vi "P9P14T_Queue_Commands.vi"(1 "P9/P14-Magnet-Control":T1 {"Approach" items=["Linear", "NoOvershoot", "Oscillate"]}, 2 "P9/P14-Magnet-Control old status":T1 {"Approach" items=["Linear", "NoOvershoot", "Oscillate"]}, 3 "16T Queue":refnum<queue>) -> (0 "P9/P14-Magnet-Control new status":T1 {"Approach" items=["Linear", "NoOvershoot", "Oscillate"]})   [LabVIEW 2019]
uses:
  PPMS/P9P14_Magnet_Control.ctl
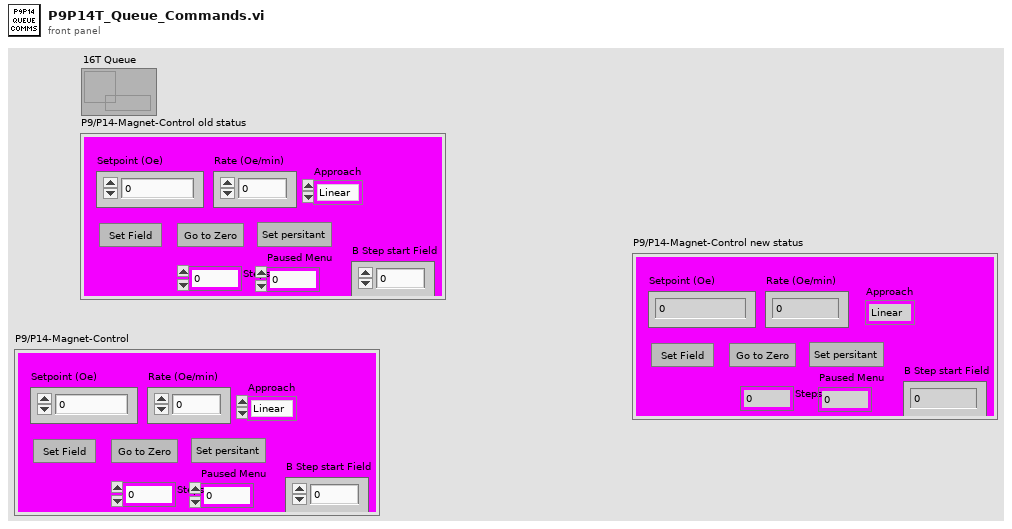
[diagram p1: front panel]
types:
  T1 = typedef "P9P14_Magnet_Control.ctl" = cluster{"Setpoint (Oe)":dbl, "Rate (Oe/min)":dbl, "Set Field":bool, "Go to zero":bool, "Set Persitant/non-pers":bool, "Approach":i32, "Steps":dbl, "Paused Menu":dbl, "B Step start Field":dbl}
  T2 = cluster{"Setpoint (Oe)":bool, "Rate (Oe/min)":bool, "Set Field":bool, "Go to zero":bool, "Set Persitant/non-pers":bool, "Approach":bool, "Steps":bool, "Paused Menu":bool, "B Step start Field":bool}
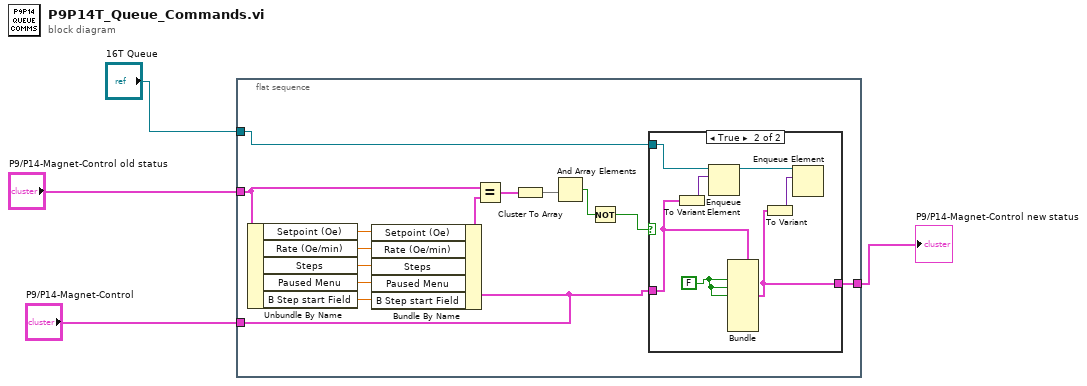
[diagram p0: block diagram]
diagram:
  n1 = flat-sequence {
    tunnel: "16T Queue" -> [w18]
    tunnel: "P9/P14-Magnet-Control old status" -> [w15]
    tunnel: "P9/P14-Magnet-Control" -> [w9]
    tunnel: [w8] -> w1
    frame #0 {
      n2 = Unbundle By Name(w15) -> ("Setpoint (Oe)"=w17:dbl, "Rate (Oe/min)"=w16:dbl, "Steps"=w7:dbl, "Paused Menu"=w6:dbl, "B Step start Field"=w5:dbl)
      n3 = Bundle By Name(cluster=w9, "Setpoint (Oe)"=w17, "Rate (Oe/min)"=w16, "Steps"=w7, "Paused Menu"=w6, "B Step start Field"=w5) -> (w14:T1)
      n4 = Equal?(x=w15, y=w14) -> (x = y?=w13:T2)
      n5 = Cluster To Array(cluster=w13) -> (array=w12:bool[])
      n6 = And Array Elements(Boolean array=w12) -> (logical AND=w11:bool)
      n7 = Not(x=w11) -> (.not. x?=w10:bool)
      n8 = case shown="True" w10 {
        tunnel: w18 -> [_ w26]
        tunnel: w9 -> [w19 w24]
        tunnel: [w19 w23] -> w8
        frame False {
        }
        frame True {
          w20 = FALSE
          n9 = To Variant(anything=w24) -> (Variant=w25:variant)
          n10 = Enqueue Element(queue=w26, element=w25) -> (queue out=w21:refnum<queue>)  [unwired: 2 in, 2 out]
          n11 = Bundle(cluster=w24, "Set Field"=w20, "Go to zero"=w20, "Set Persitant/non-pers"=w20) -> (w23:T1)  [unwired: 6 in]
          n12 = To Variant(anything=w23) -> (Variant=w22:variant)
          n13 = Enqueue Element(queue=w21, element=w22) -> ()  [unwired: 2 in, 3 out]
        }
      }
    }
  }
  "P9/P14-Magnet-Control new status" <- w1
